vi "InitializeFPGAacquisition.vi"(8 "error in (no error)":errorcluster, 11 "923x Acquisition Config":T1={"NumberOfModules"=0, "Dynamic FPGA VI Ref"=refnum, "KeyphasorX3"=[], "FixedSizeX24"={"EnabledChannels"=[], "Sensitivity"=[], "InputConfig"=[]}, "SamplingInfo"={"Number of Channels"=4, "Sampling Rate"=4.0, "Channels"=[], "Units"=[]}, "BlockSize (sec)"=0.0, "Samples To Read (per chan)"=0, "RunningAcquisitionLength"=0.0, "Settling Time"=0.0, "Waveform Groups"=[], "Acquisition Block Number"=0, "Device Name"="", "ValidConfig"=FALSE} {"FixedSizeX24"."InputConfig" items=["AC Coupled", "DC Coupled", "IEPE AC Coupled"]}) -> (0 "error out":errorcluster, 2 "start acquisition?":bool, 3 "dynamic FPGA VI reference":refnum<k20>, 4 "Sampling Rate (dbl)":dbl, 6 "Sample Rate (u32)":u32)   [LabVIEW 2015]
doc: "Initializes the acquisition of the dynamic channels with the RIO Wfm API."
uses:
  <vilib>/addons/InsightCM/Devices/Shared/AcquireBaseLoop/controls/Configuration.ctl
  <vilib>/addons/InsightCM/Devices/Shared/AcquireBaseLoop/controls/TachometerConfig.ctl
  <vilib>/addons/InsightCM/Devices/Shared/AcquireBaseLoop/controls/FixedSizeArrays.ctl
  <vilib>/LabVIEW Targets/FPGA/cRIO/shared/nicrio_ModuleControls/nicrio_cRIO-9232_ConfigModeRing.ctl
  <vilib>/addons/InsightCM/Devices/Shared/cRIOWfmAcq/subVIs/RIO Wfm Cust Ctrls/rwfm_SamplingInfo.ctl
  <vilib>/addons/InsightCM/Devices/Shared/AcquireBaseLoop/controls/Group.ctl
  <vilib>/addons/InsightCM/Devices/Shared/AcquireBaseLoop/controls/Channel.ctl
  <vilib>/addons/InsightCM/Utilities/ChannelStatus/controls/RangeParams.ctl
  <vilib>/Utility/error.llb/Error Cluster From Error Code.vi
  <vilib>/rvi/errors/niLvFpgaAdjustHostInterfaceError.vi
  <vilib>/rvi/interface/nirviReadWriteControl/nirviReadWriteControl.xnode
  <vilib>/addons/InsightCM/Devices/Shared/cRIOWfmAcq/cRIOWfmLib.lvlib
  NiFpgaLv.dll
  <vilib>/rvi/interface/Simulation/niFpgaSimulationCallBeginRW.vi
  <vilib>/addons/InsightCM/Devices/Shared/AcquireBaseLoop/FpgaAcquisition923x.lvlib
  <vilib>/addons/InsightCM/Utilities/ChannelStatus/ChannelStatus.lvlib
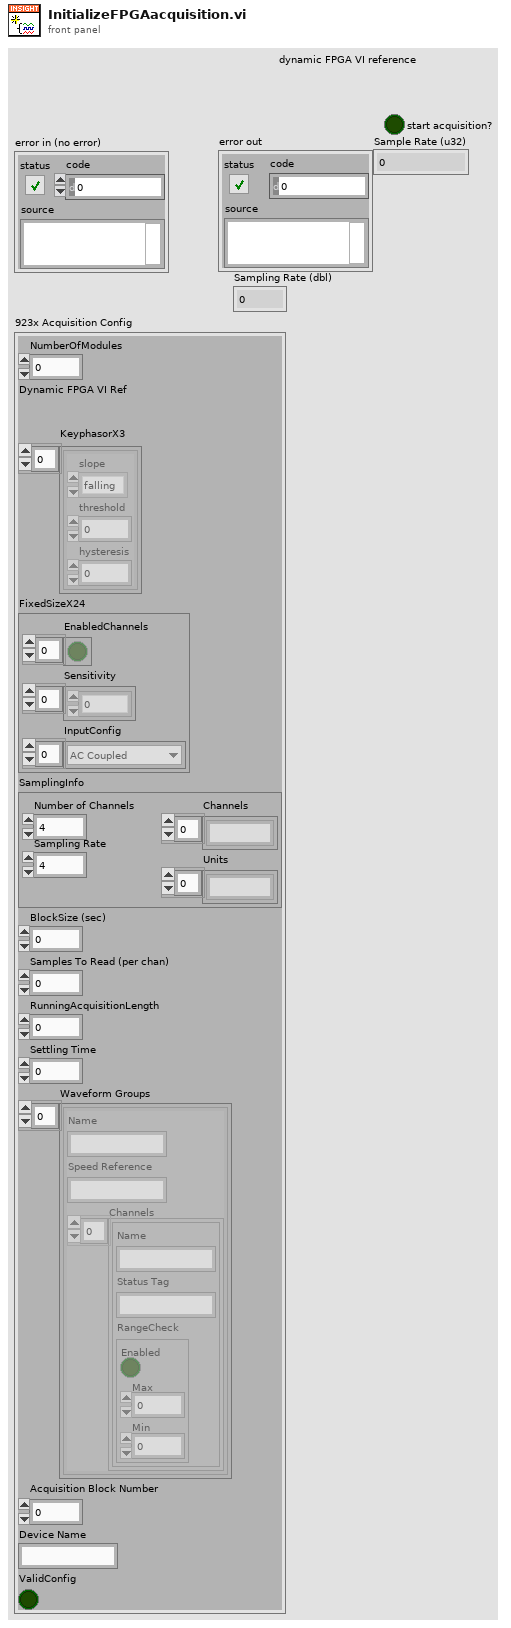
[diagram p1: front panel]
types:
  T1 = typedef "FpgaAcquisition923x.lvlib/Configuration.ctl" = cluster{"NumberOfModules":i16, "Dynamic FPGA VI Ref":refnum<k20>, "KeyphasorX3":T2[], "FixedSizeX24":T3, "SamplingInfo":T5, "BlockSize (sec)":dbl, "Samples To Read (per chan)":i32, "RunningAcquisitionLength":dbl, "Settling Time":dbl, "Waveform Groups":T6[], "Acquisition Block Number":i32, "Device Name":string, "ValidConfig":bool}
  T2 = typedef "FpgaAcquisition923x.lvlib/TachometerConfig.ctl" = cluster{"slope":enum16{"falling", "rising"}, "threshold":dbl, "hysteresis":dbl}
  T3 = typedef "FpgaAcquisition923x.lvlib/FixedSizeArrays.ctl" = cluster{"EnabledChannels":bool[], "Sensitivity":dbl[], "InputConfig":T4[]}
  T4 = typedef "nicrio_cRIO-9232_ConfigModeRing.ctl" = u8
  T5 = typedef "cRIOWfmLib.lvlib/rwfm_SamplingInfo.ctl" = cluster{"Number of Channels":i32, "Sampling Rate":dbl, "Channels":string[], "Units":string[]}
  T6 = typedef "FpgaAcquisition923x.lvlib/Group.ctl" = cluster{"Name":string, "Speed Reference":string, "Channels":T7[]}
  T7 = typedef "FpgaAcquisition923x.lvlib/Channel.ctl" = cluster{"Name":string, "Status Tag":string, "RangeCheck":T8}
  T8 = typedef "ChannelStatus.lvlib/RangeParams.ctl" = cluster{"Enabled":bool, "Max":dbl, "Min":dbl}
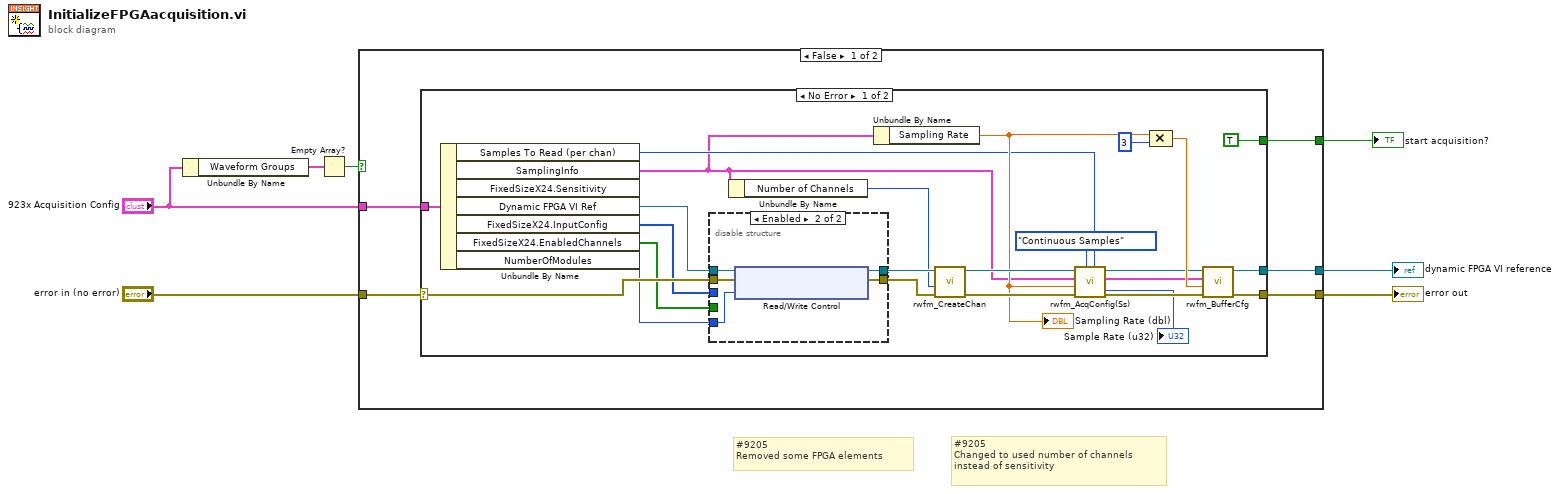
[diagram p0: block diagram]
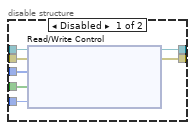
[diagram p2: hidden frame]
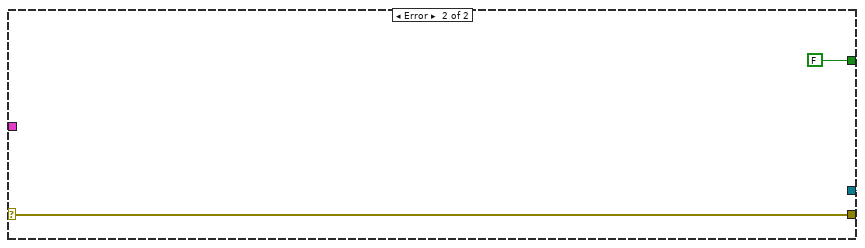
[diagram p3: hidden frame]
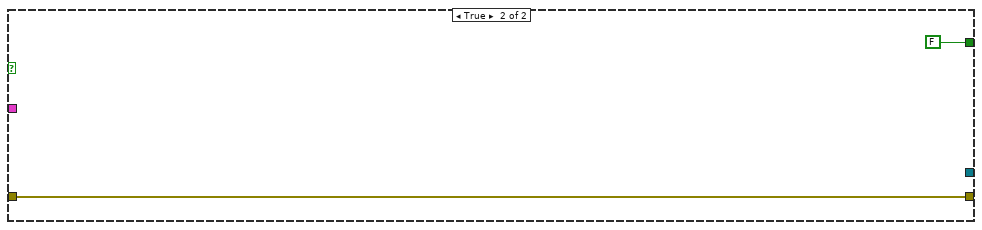
[diagram p4: hidden frame]
diagram:
  # "#9205\nChanged to used number of channels\ninstead of sensitivity"
  # "#9205\nRemoved some FPGA elements"
  n1 = Unbundle By Name("923x Acquisition Config") -> ("Waveform Groups"=w4:T6[])
  n2 = Empty Array?(array=w4) -> (empty?=w2:bool)
  n3 = case shown="False" w2 {
    tunnel: "923x Acquisition Config" -> [w12 _]
    tunnel: [w11 w53] -> w7
    tunnel: "error in (no error)" -> [w10 w53]
    tunnel: [w9 _] -> w5
    tunnel: [w8 FALSE] -> w3
    frame False {
      n4 = case shown="No Error" w10 {
        selector: w10 -> [w33 w50]
        tunnel: w12 -> [w36 _]
        tunnel: [w35 w50] -> w11
        tunnel: [w34 refnum<k0> refnum] -> w9
        tunnel: [TRUE FALSE] -> w8
        frame No Error {
          n5 = Unbundle By Name(w36) -> ("Samples To Read (per chan)"=w20:i32, "SamplingInfo"=w14:T5, "Dynamic FPGA VI Ref"=w32:refnum<k20>, "FixedSizeX24.InputConfig"=w17:T4[], "FixedSizeX24.EnabledChannels"=w18:bool[], "NumberOfModules"=w19:i16)  [unwired: 1 out]
          n6 = disable-structure shown="Enabled" {
            disable-tunnel: w33 -> [w43 w48]
            disable-tunnel: w32 -> [w42 w47]
            disable-tunnel: [w41 w46] -> w31
            disable-tunnel: [w40 w45] -> w26
            disable-tunnel: w19 -> [w39 w44]
            disable-tunnel: w18 -> [w38 _]
            disable-tunnel: w17 -> [w37 _]
            frame Disabled {
              n7 = xnode "Read/Write Control"("FPGA VI Reference In"=w42, "error in"=w43, "Input Config Array"=w37, "Enable Chan Array"=w38, "Number of Modules"=w39) -> ("FPGA VI Reference Out"=w41:refnum<k20>, "error out"=w40:errorcluster)
            }
            frame Enabled {
              n8 = xnode "Read/Write Control"("FPGA VI Reference In"=w47, "error in"=w48, "Number of Modules"=w44) -> ("FPGA VI Reference Out"=w46:refnum<k20>, "error out"=w45:errorcluster)
            }
          }
          n9 = Unbundle By Name(w14) -> ("Number of Channels"=w13:i32)
          n10 = Unbundle By Name(w14) -> ("Sampling Rate"=w21:dbl)
          "Sampling Rate (dbl)" <- w21
          n11 = call "rwfm_CreateChan.vi"("error in"=w26, "Total Avail Channels"=w13, "Dynamic FPGA VI Reference"=w31) -> ("error out"=w22:errorcluster, "Dynamic FPGA VI Reference"=w23:refnum<k20>)  [unwired: 7 in]
          n12 = call <vilib>:"rwfm_AcqConfig(Ss).vi"("Samples per Channel"=w20, "Sample Mode"=enum16{"Finite Samples", "Continuous Samples"}."Continuous Samples", "error in"=w22, "Sample Rate S/s"=w21, "Sampling Info In"=w14, "Dynamic FPGA Ref"=w23) -> ("error out"=w24:errorcluster, "Sampling Info Out"=w28:T5, "Dynamic FPGA Ref Out"=w25:refnum<k20>, "Sample Rate (u32)"=→"Sample Rate (u32)":u32)  [unwired: 1 in, 1 out]
          n13 = Compound Arithmetic op=MULTIPLY(w21, 3 ("value")) -> (w29:dbl)
          n14 = call <vilib>:"rwfm_BufferCfg.vi"("error in"=w24, "Buffer Size [Samps per Chan]"=w29, "Sampling Info In"=w28, "Dynamic FPGA VI Reference"=w25) -> ("error out"=w35:errorcluster, "Dynamic FPGA VI Reference"=w34:refnum<k20>)  [unwired: 4 in, 2 out]
        }
        frame Error {
          (unwired) cluster{"valid":bool, "description":string} {"valid"=FALSE, "description"=""} ("ConfigStatus")
        }
      }
    }
    frame True {
    }
  }
  "error out" <- w7
  "dynamic FPGA VI reference" <- w5
  "start acquisition?" <- w3
